vi "Probe cooling rate.vi"() -> ()   [LabVIEW 2020]
panel:
  in  "Temp Controller Model":T1(ring)
  out "Current \nTemperature":dbl format="%.2f"
  out "Current Rate (K/min)":dbl format="%.2f"
  in  "Desired Rate (K/min)":dbl format="%.2f"
  in  "stop":bool
  in  "seconds to wait":u32
  in  "Instrument Address":refnum<visa-resource-name>
  out "Waveform Chart":dbl[][](graph)
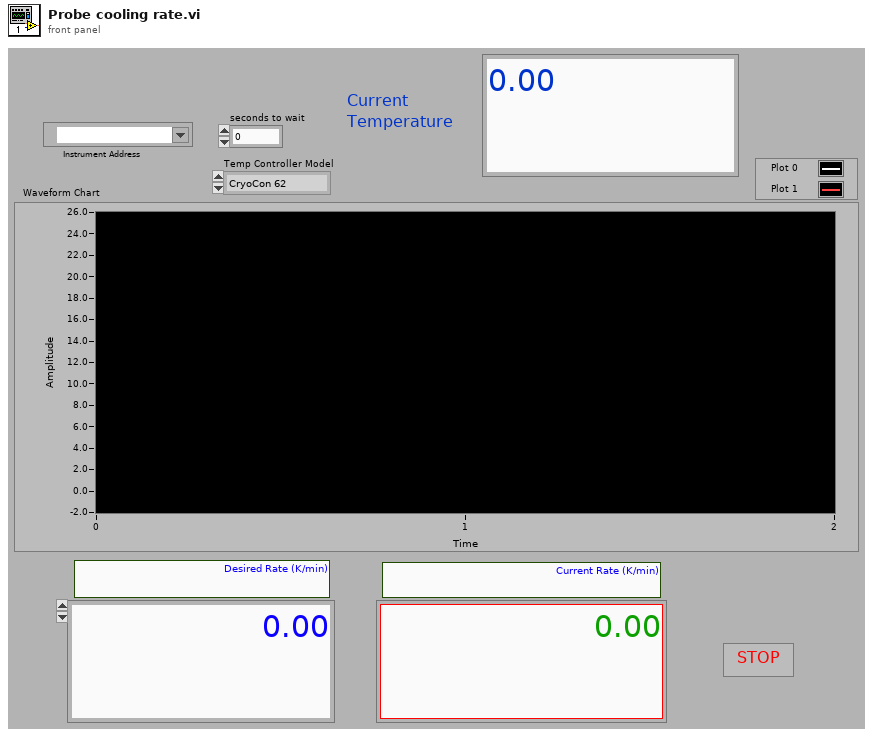
[diagram p1: front panel]
types:
  T1 = enum16{"CryoCon 62", "Conductus LTC20", "LakeShore 340"}
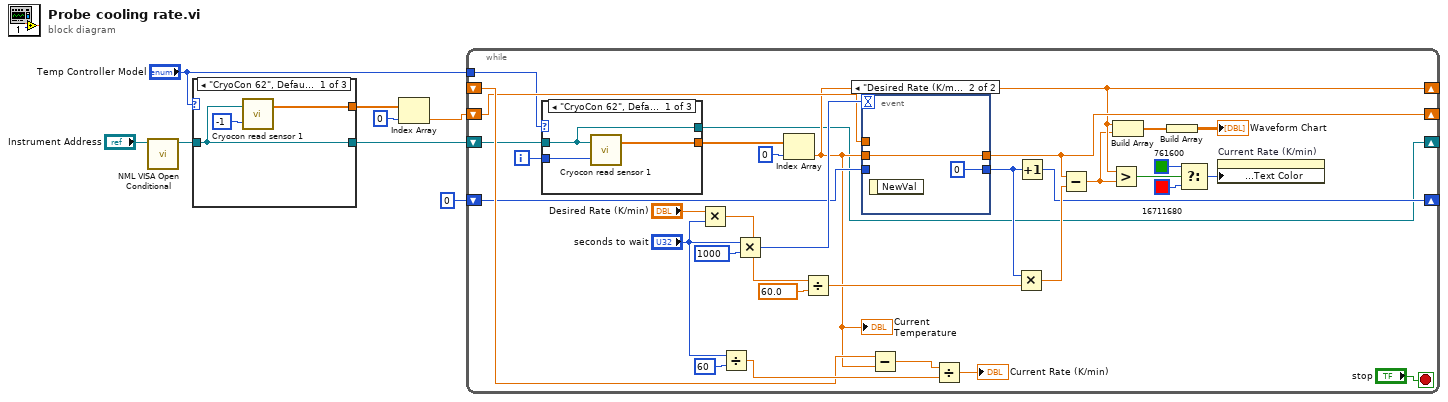
[diagram p0: block diagram]
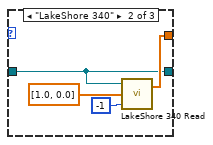
[diagram p2: hidden frame]
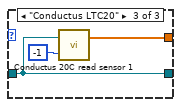
[diagram p3: hidden frame]
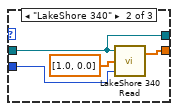
[diagram p4: hidden frame]
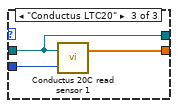
[diagram p5: hidden frame]
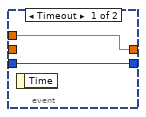
[diagram p6: hidden frame]
diagram:
  n1 = call "NML VISA Open Conditional.vi"("VISA resource name"="Instrument Address") -> ("dup VISA Session"=w1:refnum<visa-resource-name>)  [unwired: 8 in, 2 out]
  n2 = case shown="\"CryoCon 62\", Default" "Temp Controller Model" {
    tunnel: w1 -> [w9 w12 w16]
    tunnel: [w10 w15 w17] -> w8
    tunnel: [w9 w12 w16] -> w2
    frame "CryoCon 62", Default {
      n3 = call "Cryocon read sensor 1.vi"("Point #"=-1, "Instrument Address"=w9) -> ("Output"=w10:dbl[])  [unwired: 1 out]
    }
    frame "LakeShore 340" {
      n4 = call "LakeShore 340 Read.vi"("Point #"=-1, "Parameters"=dbl[] [1.0, 0.0], "Instrument Address"=w12) -> ("Measurement"=w15:dbl[])  [unwired: 1 out]
    }
    frame "Conductus LTC20" {
      n5 = call "Conductus 20C read sensor 1.vi"("Point #"=-1, "Instrument Address"=w16) -> ("Output"=w17:dbl[])  [unwired: 1 out]
    }
  }
  n6 = Index Array(array=w8, index=0) -> (element=w5:dbl)
  n7 = while {
    shift-right: [w25] -> _
    shift-left: _ -> [w38]
    shift-right: [w35] -> _
    shift-left: 0 ("counter") -> [w33]
    shift-right: [w30] -> _
    shift-left: w5 -> [w31]
    tunnel: "Temp Controller Model" -> [w20]
    shift-right: [w19] -> _
    shift-left: w2 -> [w23]
    i -> [w22]
    stop <- "stop" stop-if-true
    n8 = case shown="\"CryoCon 62\", Default" w20 {
      tunnel: w23 -> [w52 w55 w59]
      tunnel: [w54 w58 w61] -> w21
      tunnel: w22 -> [w53 w56 w60]
      tunnel: [w52 w55 w59] -> w19
      frame "CryoCon 62", Default {
        n9 = call "Cryocon read sensor 1.vi"("Point #"=w53, "Instrument Address"=w52) -> ("Output"=w54:dbl[])  [unwired: 1 out]
      }
      frame "LakeShore 340" {
        n10 = call "LakeShore 340 Read.vi"("Point #"=w56, "Parameters"=dbl[] [1.0, 0.0], "Instrument Address"=w55) -> ("Measurement"=w58:dbl[])  [unwired: 1 out]
      }
      frame "Conductus LTC20" {
        n11 = call "Conductus 20C read sensor 1.vi"("Point #"=w60, "Instrument Address"=w59) -> ("Output"=w61:dbl[])  [unwired: 1 out]
      }
    }
    n12 = Multiply(x="Desired Rate (K/min)", y="seconds to wait") -> (x*y=w49:dbl)
    n13 = Divide(x="seconds to wait", y=u32 60 ("x")) -> (x/y=w46:dbl)
    n14 = Multiply(x="seconds to wait", y=1000) -> (x*y=w43:u32)
    n15 = Index Array(array=w21, index=0) -> (element=w25:dbl)
    "Current \nTemperature" <- w25
    n16 = Divide(x=w49, y=60.0) -> (x/y=w34:dbl)
    n17 = event shown="[1] \"Desired Rate (K/min)\": Value Change" {
      selector: _ -> [_ _]
      dyn-events: _ -> [_ _]
      timeout: w43 -> [_ _]
      tunnel: w25 -> [_ w64]
      tunnel: w33 -> [w63 _]
      tunnel: [w63 0 ("counter")] -> w32
      tunnel: w31 -> [w62 _]
      tunnel: [w62 w64] -> w30
      event Timeout {
        n18 = event-data() -> ()  [unwired: 1 in, 1 out]
      }
      event "Desired Rate (K/min)": Value Change {
        n19 = event-data() -> ()  [unwired: 1 in, 1 out]
      }
    }
    n20 = Subtract(x=w38, y=w25) -> (x-y=w45:dbl)
    n21 = Divide(x=w45, y=w46) -> (x/y=→"Current Rate (K/min)":dbl)
    n22 = Multiply(x=w32, y=w34) -> (x*y=w36:dbl)
    n23 = Increment(x=w32) -> (x+1=w35:i32)
    n24 = Subtract(x=w30, y=w36) -> (x-y=w24:dbl)
    n25 = Greater?(x=w25, y=w24) -> (0:w26:bool)
    n26 = Build Array(w25, w24) -> (w40:dbl[])
    n27 = Build Array(w40) -> (→"Waveform Chart":dbl[][])
    n28 = Select(t=u32 761600, s=w26, f=u32 16711680) -> (s? t:f=w29:u32)
    n29 = property on="Current Rate (K/min)" class="DigNum (strict)"("Numeric Text.Text Colors:Text Color"=w29) -> ()  [unwired: 2 in, 2 out]
  }
